vi "parse_time_array.vi"(4 "error in":errorcluster, 5 "Array Size":i32=-1, 6 "type":cluster{"secs":i32, "nsecs":i32}[](array[cluster]), 7 "msg in":string) -> (0 "error out":errorcluster, 2 "Times":cluster{"secs":i32, "nsecs":i32}[](array[cluster]), 3 "msg out":string)   [LabVIEW 2014]
doc: "Parses out a ROS time array from msg in. The remaining string is returned in msg out.\n\nIf array size is negative, it parses a variable length array\nOtherwise it returns array of length specified."
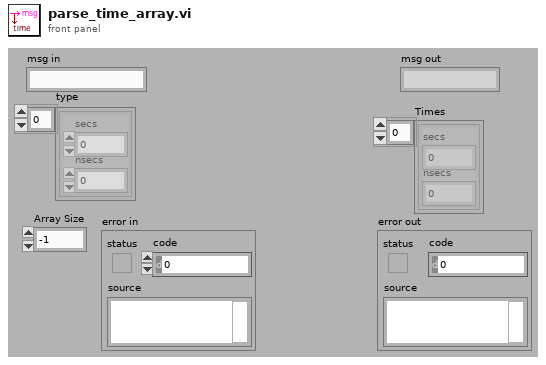
[diagram p1: front panel]
types:
  T1 = enum16{"big-endian, network order", "native, host order", "little-endian"}
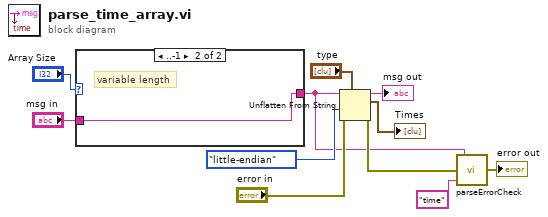
[diagram p0: block diagram]
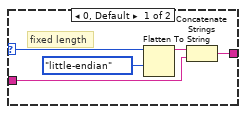
[diagram p2: hidden frame]
diagram:
  n1 = case shown="..-1" "Array Size" {
    selector: "Array Size" -> [w16 _]
    tunnel: "msg in" -> [w13 w17]
    tunnel: [w12 w17] -> w1
    frame 0, Default {
      # "fixed length"
      n2 = Flatten To String(anything=w16, byte order (0:big-endian, network order)=T1."little-endian") -> (data string=w14:string)  [unwired: 2 in, 2 out]
      n3 = Concatenate Strings(w14, w13) -> (w12:string)
    }
    frame ..-1 {
      # "variable length"
    }
  }
  n4 = Unflatten From String(type="type", binary string=w1, byte order (0:big-endian, network order)=T1."little-endian", error in (no error)="error in") -> (rest of the binary string=→"msg out":string, value=→"Times":cluster{"secs":i32, "nsecs":i32}[], error out=w5:errorcluster)  [unwired: 1 in]
  n5 = call <userlib>:"parseErrorCheck.vi"("type"="time", "error in"=w5, "msg read"=w1) -> ("error out"=→"error out":errorcluster)
